vi "Execute.vi"(6 "commandTimeout":i32=-1, 7 "CommandType":i32(ring)=-1 items=["Text"=1, "StoredProcedure"=4, "TableDirect"=512], 8 "error in (no error)":errorcluster, 9 "DynamicParameters":refnum<class "DynamicParameters.lvclass">, 10 "sql":string, 11 "SqlMapper in":refnum<class "SqlMapper.lvclass">) -> (0 "error out":errorcluster, 2 "affectedRows":i32, 3 "SqlMapper out":refnum<class "SqlMapper.lvclass">)   [LabVIEW 2020, in "ORM.lvlib" / "SqlMapper.lvclass"]
uses:
  SqlMapper.lvclass
  DynamicParameters/DynamicParameters.lvclass
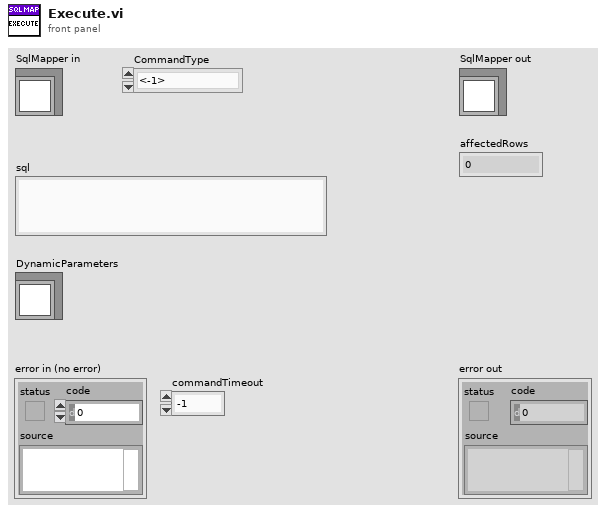
[diagram p1: front panel]
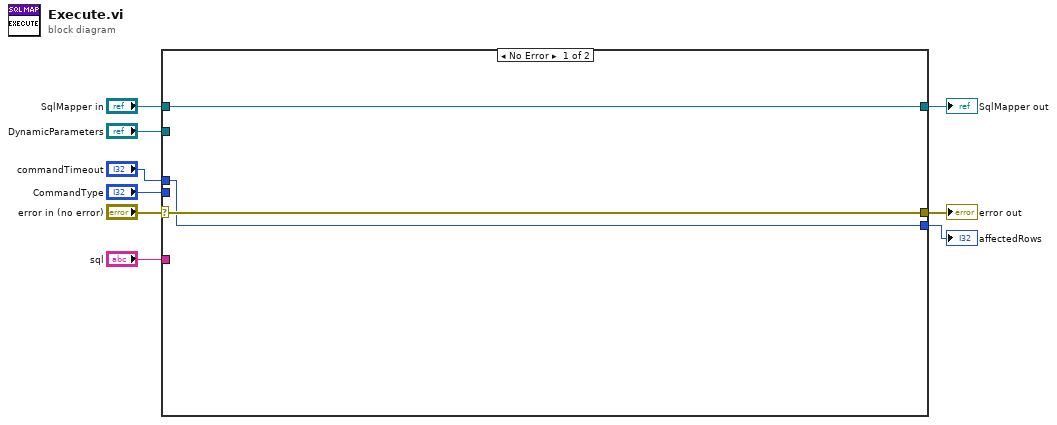
[diagram p0: block diagram]
diagram:
  n1 = case shown="No Error" "error in (no error)" {
    selector: "error in (no error)" -> [w12 w14]
    tunnel: [w12 w14] -> w8
    tunnel: [w11 w13] -> w6
    tunnel: "SqlMapper in" -> [w11 w13]
    tunnel: "sql" -> [_ _]
    tunnel: "CommandType" -> [_ _]
    tunnel: "DynamicParameters" -> [_ _]
    tunnel: [w10 _] -> w2
    tunnel: "commandTimeout" -> [w10 _]
    frame No Error {
    }
    frame Error {
    }
  }
  "error out" <- w8
  "SqlMapper out" <- w6
  "affectedRows" <- w2
